vi "menu-AddMenuGroups.vi"(7 "Menu Name":string[](array[string]), 11 "element":T1[](array[typedef])) -> (3 "Array":T1[](array[typedef]))   [LabVIEW 2019]
uses:
  <resource>/Framework/Providers/API/mxLvMenuItem.ctl
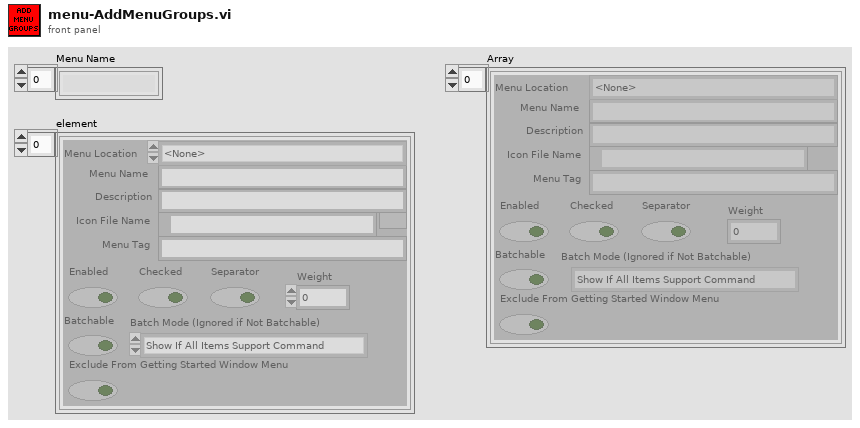
[diagram p1: front panel]
types:
  T1 = typedef "mxLvMenuItem.ctl" = cluster{"Menu Name":string, "Description":string, "Icon File Name":path, "Menu Tag":string, "Enabled":bool, "Checked":bool, "Separator":bool, "Batchable":bool, "Weight":i32, "Batch Mode (Ignored if Not Batchable)":enum32{"Show If All Items Support Command", "Show If Any Items Support Command"}, "Menu Location":enum32{"<None>", "Project", "Project / Build Specifications", "Tools", "Tools / Source Control", "Tools / Real-Time Module", "Help"}, "Exclude From Getting Started Window Menu":bool}
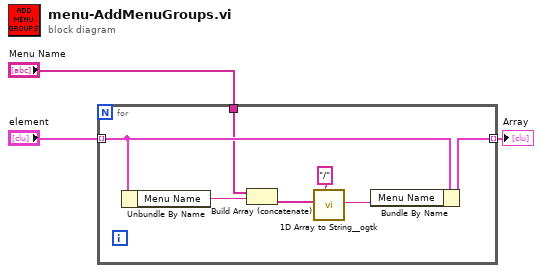
[diagram p0: block diagram]
diagram:
  n1 = for {
    tunnel: "element" -> [w9] mode=indexing
    tunnel: [w10] -> w2 mode=indexing
    tunnel: "Menu Name" -> [w7]
    n2 = Unbundle By Name(w9) -> ("Menu Name"=w4:string)
    n3 = Build Array (concatenate)(w7, w4) -> (w8:string[])
    n4 = call <userlib>:"1D Array to String__ogtk.vi"("delimiter (Tab)"="/", "Array of Strings"=w8) -> ("delimited string"=w6:string)  [unwired: 9 in]
    n5 = Bundle By Name(cluster=w9, "Menu Name"=w6) -> (w10:T1)
  }
  "Array" <- w2
